vi "MeasurementItems_GetChannelDimension.vi"(8 "error in (no error)":errorcluster, 10 "#Channel":u16, 11 "OXY_SCPI Reseource In":refnum<visa-resource-name>) -> (0 "error out":errorcluster, 1 "communication_data":T1, 2 "Range":string, 3 "OXY_SCPI Reseource Out":refnum<visa-resource-name>)   [LabVIEW 2018, in "OXYGEN.lvlib"]
doc: "Queries the dimension of the data to be transferred for one item."
uses:
  OXYGEN.lvlib
  TypeDefs/Cluster_RawCommData.ctl
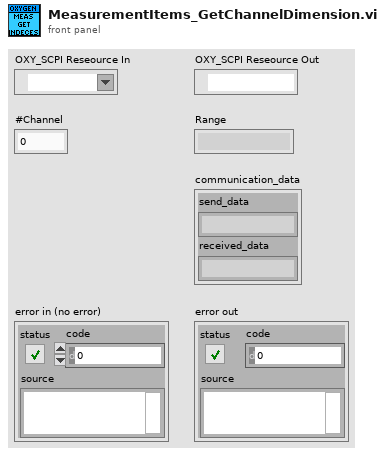
[diagram p1: front panel]
types:
  T1 = typedef "OXYGEN.lvlib/Cluster_RawCommData.ctl" = cluster{"send_data":string, "received_data":string}
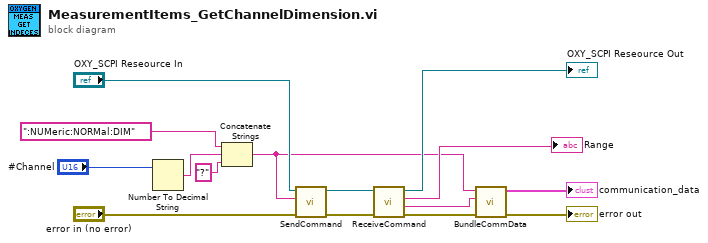
[diagram p0: block diagram]
diagram:
  n1 = Number To Decimal String(number="#Channel") -> (decimal integer string=w3:string)  [unwired: 1 in]
  n2 = Concatenate Strings(":NUMeric:NORMal:DIM" ("String to Send"), w3, "?" ("string")) -> (w1:string)
  n3 = call "SendCommand.vi"("error in (no error)"="error in (no error)", "String to Send"=w1, "OXY_SCPI Reseource In"="OXY_SCPI Reseource In") -> ("error out"=w15:errorcluster, "OXY_SCPI Reseource Out"=w14:refnum<visa-resource-name>)  [unwired: 7 in]
  n4 = call "ReceiveCommand.vi"("error in (no error)"=w15, "OXY_SCPI Reseource In"=w14) -> ("error out"=w9:errorcluster, "received Data with Header"=w7:string, "received Data"=→"Range":string, "OXY_SCPI Reseource Out"=→"OXY_SCPI Reseource Out":refnum<visa-resource-name>)  [unwired: 6 in]
  n5 = call "BundleCommData.vi"("error in (no error)"=w9, "received_data"=w7, "send_data"=w1) -> ("error out"=→"error out":errorcluster, "communication_data"=→"communication_data":T1)  [unwired: 7 in]
